vi "Read Full Rotated Buffer.vi"(8 "error in (no error)":errorcluster, 11 "Ring buffer DVR in":refnum<data-value>) -> (0 "error out":errorcluster, 1 "Values":u8[](array[numeric]), 2 "Timestamps":u64[](array[numeric]), 3 "Ring buffer DVR out":refnum<data-value>, 4 "empty buffer?":bool, 5 "#bytes per timestamp":i32)   [LabVIEW 2021, in "Ring Buffer Time Series Data.lvlib"]
uses:
  Ring Buffer Time Series Data.lvlib
  SubVIs/DVR data.ctl
  SubVIs/Split Values Array.vi
  SubVIs/Enforce array size multiple timestamps.vi
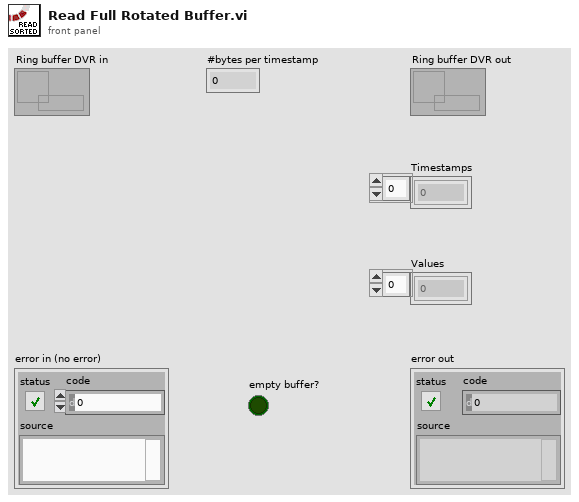
[diagram p1: front panel]
types:
  T1 = typedef "Ring Buffer Time Series Data.lvlib/DVR data.ctl" = cluster{"Timestamps":u64[], "Values":u8[], "#bytes per timestamp":i32, "Index":i32, "Size (#timestamps)":i32, "Full?":bool}
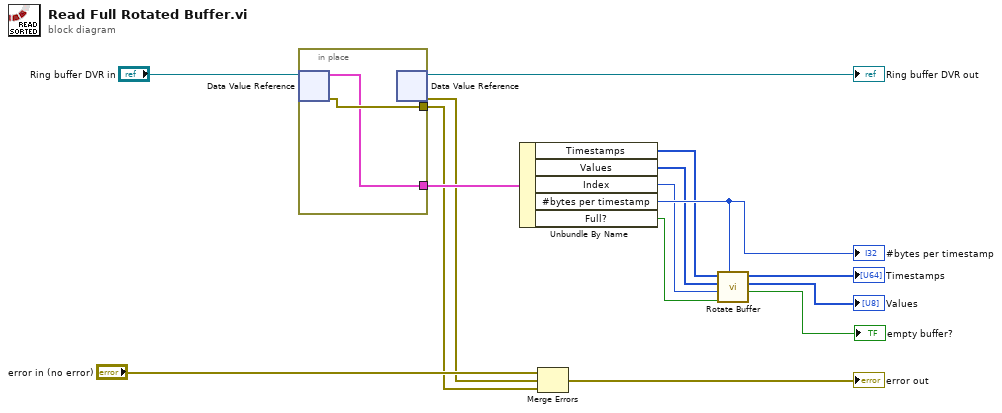
[diagram p0: block diagram]
diagram:
  n1 = in-place {
    in-place-border: [w17] -> w2
    in-place-border: [w16] -> w9
    n2 = in-place-dvr #1("Ring buffer DVR in") -> (w16:T1, w17:errorcluster)
    n3 = in-place-dvr #1() -> (→"Ring buffer DVR out":refnum<data-value>, w3:errorcluster)  [unwired: 1 in]
  }
  n4 = Unbundle By Name(w9) -> ("Timestamps"=w8:u64[], "Values"=w7:u8[], "Index"=w6:i32, "#bytes per timestamp"=w11:i32, "Full?"=w5:bool)
  "#bytes per timestamp" <- w11
  n5 = Merge Errors("error in (no error)", w3, w2) -> (→"error out":errorcluster)
  n6 = call "Rotate Buffer.vi"("#bytes per value"=w11, "Full?"=w5, "Index"=w6, "Values"=w7, "Timestamps"=w8) -> ("empty buffer?"=→"empty buffer?":bool, "Values"=→"Values":u8[], "Timestamps"=→"Timestamps":u64[])  [unwired: 4 in]
